vi "CS_cRIO-PB_MSAC2_DPV1-AbortReq.vi"(0 "FPGA VI Reference":T3, 5 "Slave":i8, 7 "Abort data":T4 {"Additional detail:" format="%04x"; "Instance &\nReasoncode:" format="%.0x"; "Subnet:" format="%0.0f"; "Communication ref.:" format="%0.0f"}, 11 "Error":errorcluster) -> (4 "FPGA VI Reference out":T3, 6 "Result":T2, 8 "Abort data":T1 {"Reasoncode:" format="%.0x"; "Instance:" format="%.0x"; "Additional detail:" format="%04x"; "Subnet:" format="%.0x"; "Response SAP:" format="%0.0f"; "Remote address:" format="%0.0f"}, 15 "Error out":errorcluster)   [LabVIEW 2013, in "dynamic profibus.lvlib"]
doc: "Handles the cyclic process data of the selected DP-Slave.\n\nFPGA VI Reference:\nReference of the FPGA VI.\n\nSlave:\nPROFIBUS address of the DP-Slave. \n\nModify output data:\nThe Modify output data array contains the DP-Slave output data to be changed.\n\nInput data:\nThe Input data array contains the DP-Slave input data.\n\nOutput data:\nThe Output data array contains the DP-Slave output data.\n\nInput length:\nReturns the configured input length of the DP-Slave.\n\nOutput length:\nReturns the configured output length of the DP-Slave.\n\nSlave status:\n0x00: DP-Slave is in DataExchange mode, input and output data are valid\n0xC3: DP-Slave is not in Data Exchange mode, input and output data are invalid, DP-Slave diagnostic data are reported in Diag data array\n0xFF: DP-Slave is in Data Exchange mode and reports ext. diagnostic data, input and output data are valid.\n\nFPGA VI Reference out:\nIs a copy of the FPGA VI Reference .\n\nError in:\nPreceding error conditions. If an error has already occurred, the VI returns the value of the error in Error out.\n\nError out:\nError: TRUE if an error occurred.\nStatus: Error code\nInfo: Error description"
uses:
  dynamic profibus.lvlib
  CS_cRIO-PB_DP-Master_FPGA-Reference.ctl
  Examples/SubVIs/CS_PB_DPV1_Result.ctl
  Examples/SubVIs/CS_PB_DPV1_AbortReqData.ctl
  Examples/SubVIs/CS_PB_DPV1_AbortIndData.ctl
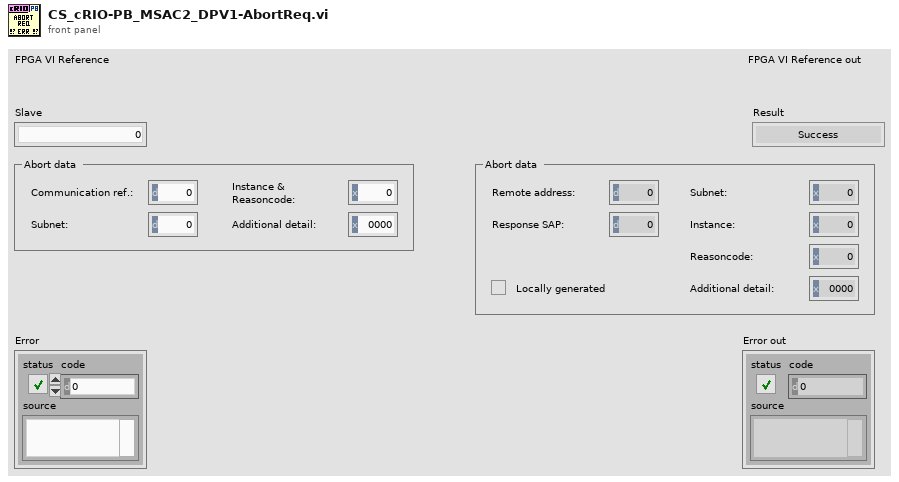
[diagram p1: front panel]
types:
  T1 = typedef "CS_PB_DPV1_AbortIndData.ctl" = cluster{"Remote address:":u8, "Response SAP:":u8, "Locally generated":bool, "Subnet:":u8, "Instance:":u8, "Reasoncode:":u8, "Additional detail:":u16}
  T2 = typedef "CS_PB_DPV1_Result.ctl" = enum16{"Success", "Abort", "Error"}
  T3 = typedef "dynamic profibus.lvlib/CS_cRIO-PB_DP-Master_FPGA-Reference.ctl" = refnum<k20>
  T4 = typedef "CS_PB_DPV1_AbortReqData.ctl" = cluster{"Communication ref.:":u8, "Subnet:":u8, "Instance &\nReasoncode:":u8, "Additional detail:":u16}
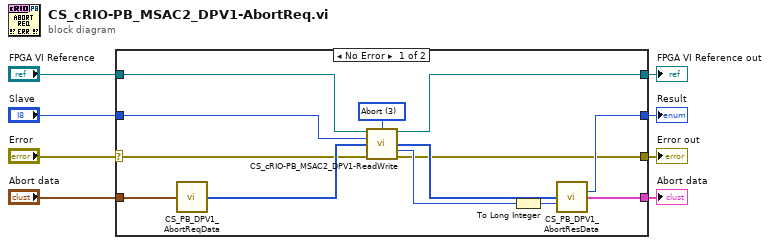
[diagram p0: block diagram]
diagram:
  n1 = case shown="No Error" "Error" {
    selector: "Error" -> [w16 w22]
    tunnel: "Slave" -> [w12 _]
    tunnel: "FPGA VI Reference" -> [w14 w23]
    tunnel: [w15 w23] -> w1
    tunnel: [w17 w22] -> w3
    tunnel: [w11 _] -> w4
    tunnel: [w19 _] -> w2
    tunnel: "Abort data" -> [w9 _]
    frame No Error {
      w13 = i8 3 items=["Initiate", "Read", "Write", "Abort"] ("DPV1-Service")
      n2 = call "CS_PB_DPV1_AbortReqData.vi"("Abort data"=w9) -> ("Request data"=w20:u8[])  [unwired: 14 in]
      n3 = call "CS_cRIO-PB_MSAC2_DPV1-ReadWrite.vi"("FPGA VI Reference"=w14, "DPV1-Service"=w13, "Slave"=w12, "Data"=w20, "Error"=w16) -> ("FPGA VI Reference out"=w15:T3, "Data out"=w21:u8[], "Status"=w18:u8, "Error out"=w17:errorcluster)  [unwired: 7 in]
      n4 = To Long Integer(number=w18) -> (32bit integer=w10:i32)
      n5 = call "CS_PB_DPV1_AbortResData.vi"("Response data"=w21, "Status"=w10) -> ("Result"=w19:T2, "Abort data"=w11:T1)  [unwired: 12 in]
    }
    frame Error {
    }
  }
  "Error out" <- w3
  "FPGA VI Reference out" <- w1
  "Result" <- w2
  "Abort data" <- w4
